vi "OnResume.vi"(8 "error in (no error)":errorcluster, 10 "Engine in":refnum<class "Engine.lvclass">, 11 "Bouncer in":refnum<class "Bouncer.lvclass">) -> (0 "error out":errorcluster, 2 "Engine out":refnum<class "Engine.lvclass">, 3 "Bouncer out":refnum<class "Bouncer.lvclass">)   [LabVIEW 2019, in "RT_Game.lvlib" / "Bouncer.lvclass"]
uses:
  Bouncer.lvclass
  C:/Users/FreshBob/Dropbox/VIs/myRIO_GameConsole/RT/RT_Game/Game/Game.lvclass
  Engine/Engine.lvclass
  Menu/States.ctl
  Game/Game.lvclass/Game.ctl
  Game/Read Singleplayer.vi
  Game/Read SingleplayerBeforeMenu.vi
  Game/Read StateBeforeMenu.vi
  Game/Write State.vi
  Game/Game.lvclass
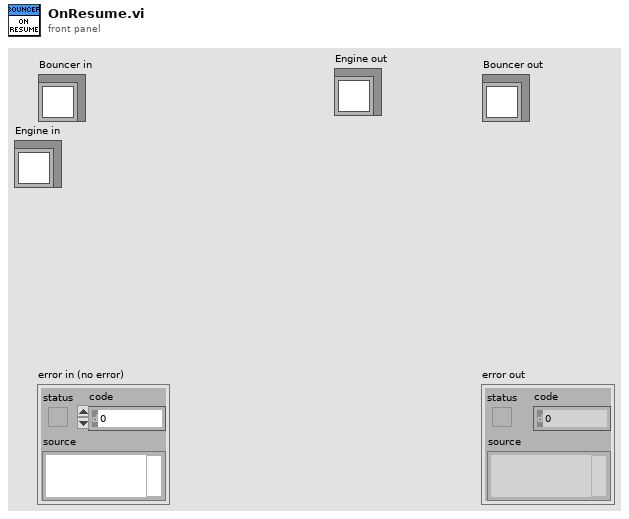
[diagram p1: front panel]
types:
  T1 = typedef "RT_Game.lvlib/Game.lvclass/States.ctl" = enum16{"Init", "Restart", "Menu", "Game", "Resume", "ToggleSingleplayer", "LoadNextGame", "ExitToMenu", "NewHighscore", "GameOver", "SlideOut", "FadeToMenu", "StartFadeToMenu"}
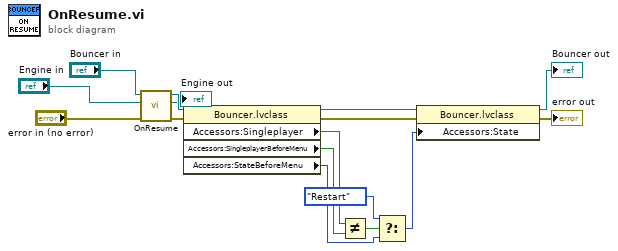
[diagram p0: block diagram]
diagram:
  n1 = call-parent "OnResume.vi"("error in (no error)"="error in (no error)", "Engine in"="Engine in", "Game in"="Bouncer in") -> ("error out"=w16:errorcluster, "Engine out"=→"Engine out":refnum<class "Engine.lvclass">, "Game out"=w12:refnum<class "Bouncer.lvclass">)  [unwired: 6 in]
  n2 = property class="Bouncer.lvclass"(reference=w12, error in=w16) -> (reference out=w8:refnum<class "Bouncer.lvclass">, error out=w13:errorcluster, "Accessors:Singleplayer"=w11:bool, "Accessors:SingleplayerBeforeMenu"=w10:bool, "Accessors:StateBeforeMenu"=w3:T1)
  n3 = Not Equal?(x=w11, y=w10) -> (x != y?=w5:bool)
  n4 = Select(t=States."Restart", s=w5, f=w3) -> (s? t:f=w7:T1)
  n5 = property class="Bouncer.lvclass"(reference=w8, error in=w13, "Accessors:State"=w7) -> (reference out=→"Bouncer out":refnum<class "Bouncer.lvclass">, error out=→"error out":errorcluster)
